vi "createSubDataEvents.vi"(8 "error in (no error)":errorcluster, 11 "DataListenerThisComponent in":refnum<class "DataListenerThisComponent.lvclass">) -> (0 "error out":errorcluster, 3 "DataListenerThisComponent out":refnum<class "DataListenerThisComponent.lvclass">)   [LabVIEW 2015]
uses:
  DataListenerThisComponent.lvclass
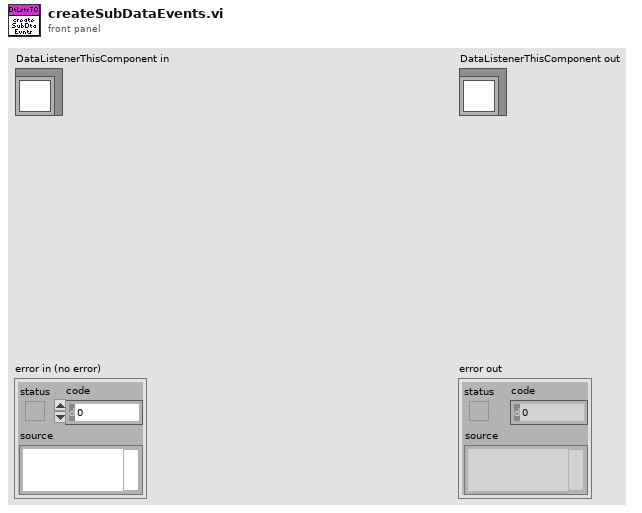
[diagram p1: front panel]
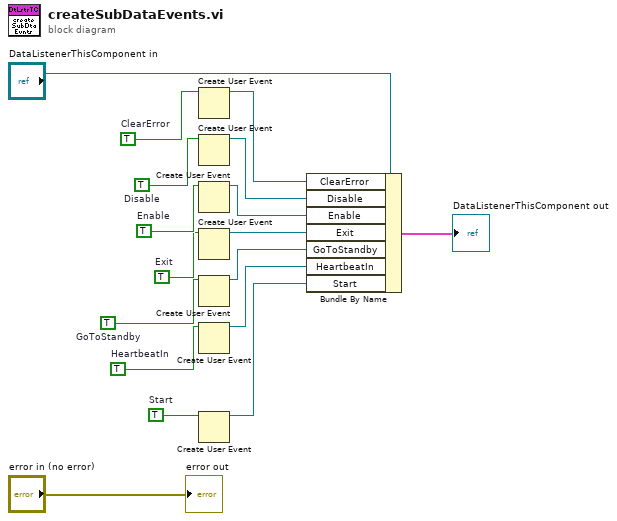
[diagram p0: block diagram]
diagram:
  w10 = TRUE  # Start
  w11 = TRUE  # HeartbeatIn
  w12 = TRUE  # GoToStandby
  w13 = TRUE  # Exit
  w14 = TRUE  # Enable
  w15 = TRUE  # Disable
  w16 = TRUE  # ClearError
  n1 = Create User Event(user event datatype=w16) -> (user event=w9:refnum<user-event>)  [unwired: 1 in, 1 out]
  n2 = Create User Event(user event datatype=w15) -> (user event=w8:refnum<user-event>)  [unwired: 1 in, 1 out]
  n3 = Create User Event(user event datatype=w14) -> (user event=w7:refnum<user-event>)  [unwired: 1 in, 1 out]
  n4 = Create User Event(user event datatype=w13) -> (user event=w6:refnum<user-event>)  [unwired: 1 in, 1 out]
  n5 = Create User Event(user event datatype=w12) -> (user event=w5:refnum<user-event>)  [unwired: 1 in, 1 out]
  n6 = Create User Event(user event datatype=w11) -> (user event=w4:refnum<user-event>)  [unwired: 1 in, 1 out]
  n7 = Create User Event(user event datatype=w10) -> (user event=w3:refnum<user-event>)  [unwired: 1 in, 1 out]
  n8 = Bundle By Name(cluster="DataListenerThisComponent in", "ClearError"=w9, "Disable"=w8, "Enable"=w7, "Exit"=w6, "GoToStandby"=w5, "HeartbeatIn"=w4, "Start"=w3) -> (→"DataListenerThisComponent out":cluster{})
  "error out" <- "error in (no error)"
